vi "UI_Move Console.vi"(8 "error in (no error)":errorcluster, 11 "UI_Move in":refnum<class "UI_Move.lvclass">) -> (0 "error out":errorcluster, 3 "UI_Move out":refnum<class "UI_Move.lvclass">)   [LabVIEW 2015, in "UI_Move.lvclass"]
uses:
  UI_Move.lvclass
panel:
  in  "Pane":refnum<vi>
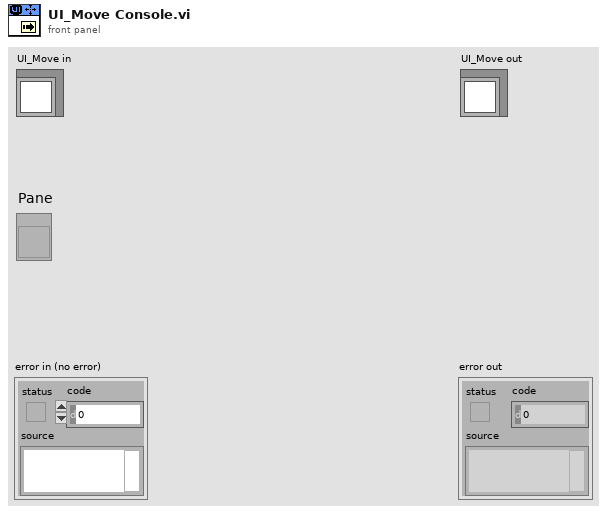
[diagram p1: front panel]
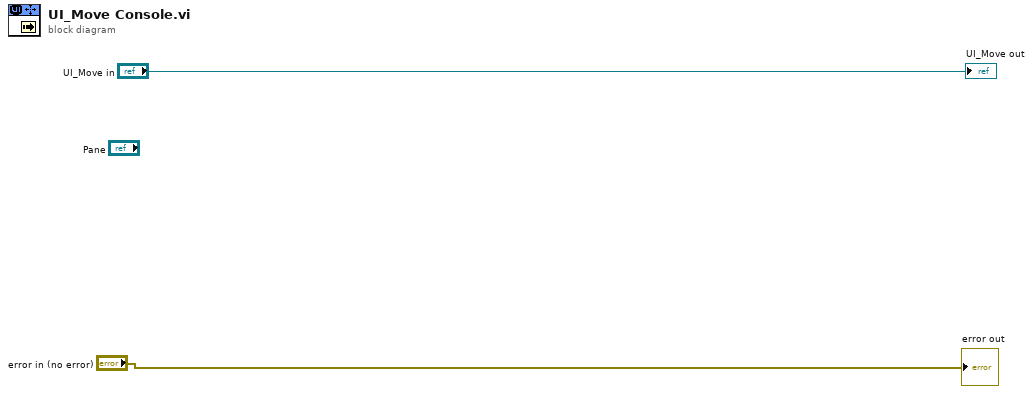
[diagram p0: block diagram]
diagram:
  "error out" <- "error in (no error)"
  "UI_Move out" <- "UI_Move in"
